vi "NI VeriStand - Close Engine State Change Notification.vi"(8 "error in (no error)":errorcluster, 10 "SystemStateRefs":T1) -> (0 "error out":errorcluster)   [LabVIEW 2020, in "NI_VS Workspace ExecutionAPI.lvlib"]
doc: "Destroys the user event created by the Open Engine State Change Notification VI."
uses:
  <vilib>/NI VeriStand/Execution/Workspace/NI_VS Workspace ExecutionAPI.lvlib
  <vilib>/NI VeriStand/Execution/Workspace/SystemStateEventRef.ctl
  <vilib>/NI VeriStand/Execution/Workspace/Target State Info.ctl
  <vilib>/NI VeriStand/Execution/Workspace/Target State.ctl
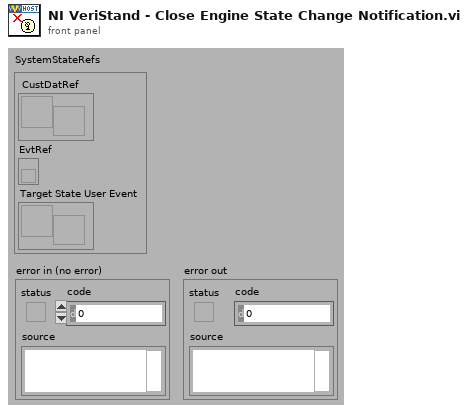
[diagram p1: front panel]
types:
  T1 = typedef "NI_VS Workspace ExecutionAPI.lvlib/SystemStateEventRef.ctl" = cluster{"CustDatRef":refnum<user-event>, "EvtRef":refnum<k27>, "Target State User Event":refnum<user-event>}
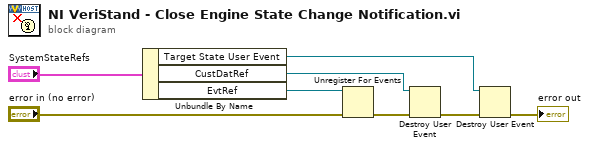
[diagram p0: block diagram]
diagram:
  n1 = Unbundle By Name("SystemStateRefs") -> ("Target State User Event"=w2:refnum<user-event>, "CustDatRef"=w4:refnum<user-event>, "EvtRef"=w7:refnum<k27>)
  n2 = Unregister For Events(event registration refnum=w7, error in="error in (no error)") -> (error out=w6:errorcluster)
  n3 = Destroy User Event(user event=w4, error in=w6) -> (error out=w3:errorcluster)
  n4 = Destroy User Event(user event=w2, error in=w3) -> (error out=→"error out":errorcluster)
